vi "Velocity Profile 2string.vi"(5 "VelocityProfiles":T1[](array[typedef])) -> (2 "VPL":string)   [LabVIEW 2014]
uses:
  PBFAM/Controller/MachineController/Converters/ScanSub/VelocityProfile.ctl
panel:
  out "VelocityProfile":T1
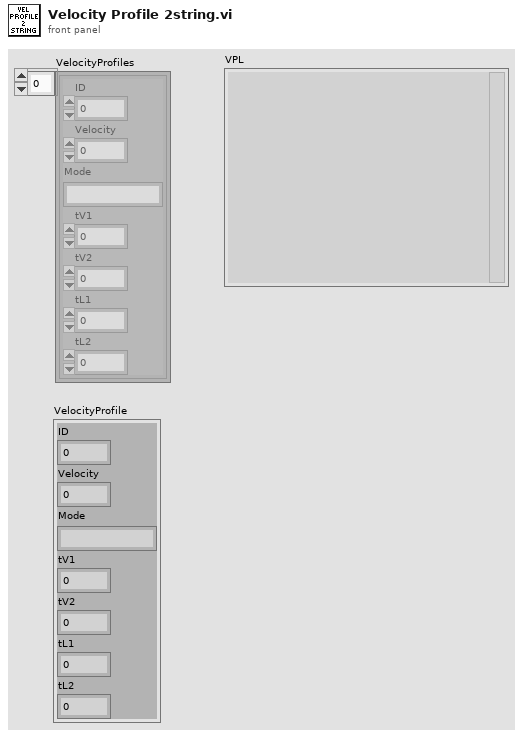
[diagram p1: front panel]
types:
  T1 = typedef "VelocityProfile.ctl" = cluster{"ID":u32, "Velocity":dbl, "Mode":string, "tV1":u32, "tV2":u32, "tL1":u32, "tL2":u32}
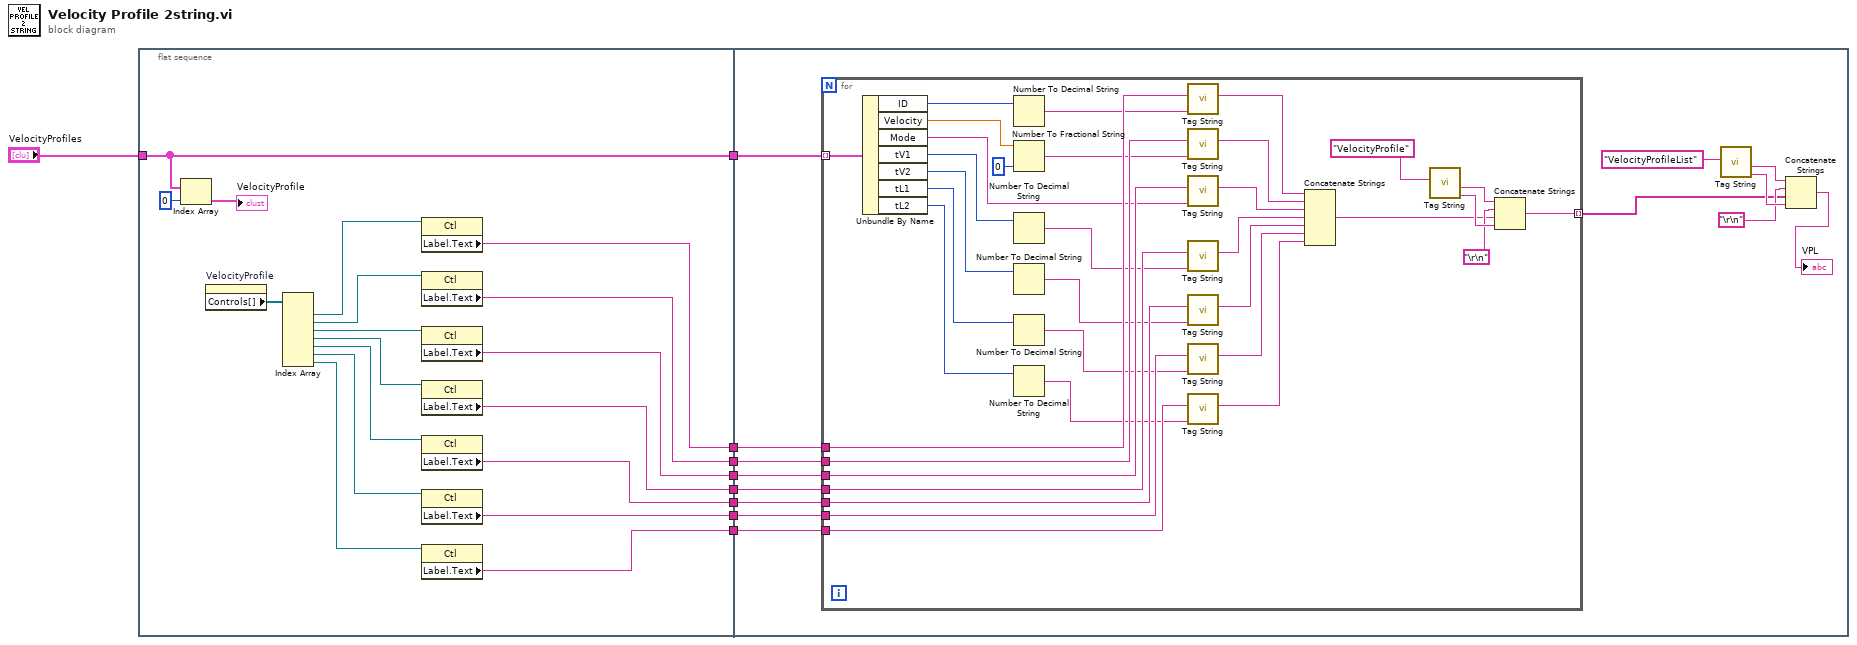
[diagram p0: block diagram]
diagram:
  n1 = flat-sequence {
    tunnel: "VelocityProfiles" -> [w26]
    tunnel: [w26] -> w8
    tunnel: [w16] -> w7
    tunnel: [w15] -> w6
    tunnel: [w14] -> w5
    tunnel: [w13] -> w4
    tunnel: [w12] -> w3
    tunnel: [w11] -> w2
    tunnel: [w10] -> w1
    tunnel: w8 -> [w41]
    tunnel: w7 -> [w40]
    tunnel: w6 -> [w39]
    tunnel: w5 -> [w38]
    tunnel: w4 -> [w37]
    tunnel: w3 -> [w36]
    tunnel: w2 -> [w35]
    tunnel: w1 -> [w34]
    frame #0 {
      n2 = Index Array(array=w26, index=0) -> (element=→"VelocityProfile":T1)
      n3 = property on="VelocityProfile" class="Clust (strict)"() -> ("Controls[]"=w27:refnum<vi>[])  [unwired: 2 in, 2 out]
      n4 = Index Array(array=w27) -> (element #1=w23:refnum<vi>, element #2=w22:refnum<vi>, element #3=w21:refnum<vi>, element #4=w20:refnum<vi>, element #5=w19:refnum<vi>, element #6=w18:refnum<vi>, element #7=w17:refnum<vi>)  [unwired: 7 in]
      n5 = property class="Ctl"(reference=w23) -> ("Label.Text"=w16:string)  [unwired: 1 in, 2 out]
      n6 = property class="Ctl"(reference=w22) -> ("Label.Text"=w15:string)  [unwired: 1 in, 2 out]
      n7 = property class="Ctl"(reference=w21) -> ("Label.Text"=w14:string)  [unwired: 1 in, 2 out]
      n8 = property class="Ctl"(reference=w20) -> ("Label.Text"=w13:string)  [unwired: 1 in, 2 out]
      n9 = property class="Ctl"(reference=w19) -> ("Label.Text"=w12:string)  [unwired: 1 in, 2 out]
      n10 = property class="Ctl"(reference=w18) -> ("Label.Text"=w11:string)  [unwired: 1 in, 2 out]
      n11 = property class="Ctl"(reference=w17) -> ("Label.Text"=w10:string)  [unwired: 1 in, 2 out]
    }
    frame #1 {
      n12 = for {
        tunnel: w41 -> [w76] mode=indexing
        tunnel: w40 -> [w69]
        tunnel: w39 -> [w67]
        tunnel: w38 -> [w65]
        tunnel: w37 -> [w63]
        tunnel: w36 -> [w61]
        tunnel: w35 -> [w59]
        tunnel: w34 -> [w57]
        tunnel: [w43] -> w28 mode=indexing
        n13 = Unbundle By Name(w76) -> ("ID"=w75:u32, "Velocity"=w74:dbl, "Mode"=w64:string, "tV1"=w73:u32, "tV2"=w70:u32, "tL1"=w71:u32, "tL2"=w72:u32)
        n14 = Number To Decimal String(number=w75) -> (decimal integer string=w68:string)  [unwired: 1 in]
        n15 = Number To Fractional String(number=w74, precision (6)=i16 0) -> (F-format string=w66:string)  [unwired: 2 in]
        n16 = Number To Decimal String(number=w73) -> (decimal integer string=w62:string)  [unwired: 1 in]
        n17 = Number To Decimal String(number=w70) -> (decimal integer string=w60:string)  [unwired: 1 in]
        n18 = Number To Decimal String(number=w71) -> (decimal integer string=w58:string)  [unwired: 1 in]
        n19 = Number To Decimal String(number=w72) -> (decimal integer string=w56:string)  [unwired: 1 in]
        n20 = call "Tag String.vi"("String In"=w68, "String name"=w69) -> ("Start Tagged String Out"=w55:string)  [unwired: 3 in, 2 out]
        n21 = call "Tag String.vi"("String In"=w66, "String name"=w67) -> ("Start Tagged String Out"=w54:string)  [unwired: 3 in, 2 out]
        n22 = call "Tag String.vi"("String In"=w64, "String name"=w65) -> ("Start Tagged String Out"=w53:string)  [unwired: 3 in, 2 out]
        n23 = call "Tag String.vi"("String In"=w62, "String name"=w63) -> ("Start Tagged String Out"=w52:string)  [unwired: 3 in, 2 out]
        n24 = call "Tag String.vi"("String In"=w60, "String name"=w61) -> ("Start Tagged String Out"=w51:string)  [unwired: 3 in, 2 out]
        n25 = call "Tag String.vi"("String In"=w58, "String name"=w59) -> ("Start Tagged String Out"=w50:string)  [unwired: 3 in, 2 out]
        n26 = call "Tag String.vi"("String In"=w56, "String name"=w57) -> ("Start Tagged String Out"=w49:string)  [unwired: 3 in, 2 out]
        n27 = Concatenate Strings(w55, w54, w53, w52, w51, w50, w49) -> (w44:string)
        n28 = call "Tag String.vi"("String name"="VelocityProfile") -> ("Stop"=w48:string, "Start"=w47:string)  [unwired: 4 in, 1 out]
        n29 = Concatenate Strings(w47, "\r\n", w44, w48) -> (w43:string)
      }
      n30 = call "Tag String.vi"("String name"="VelocityProfileList") -> ("Stop"=w32:string, "Start"=w30:string)  [unwired: 4 in, 1 out]
      n31 = Concatenate Strings(w30, "\r\n", w28, w32) -> (→"VPL":string)
    }
  }
